vi "KeepWarm.vi"() -> ()   [LabVIEW 2010]
panel:
  in  "Current (mA)":dbl
  out "Dummy":string
  in  "Laser GPIB":u8=10 max=100
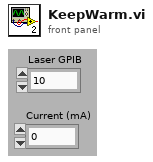
[diagram p1: front panel]
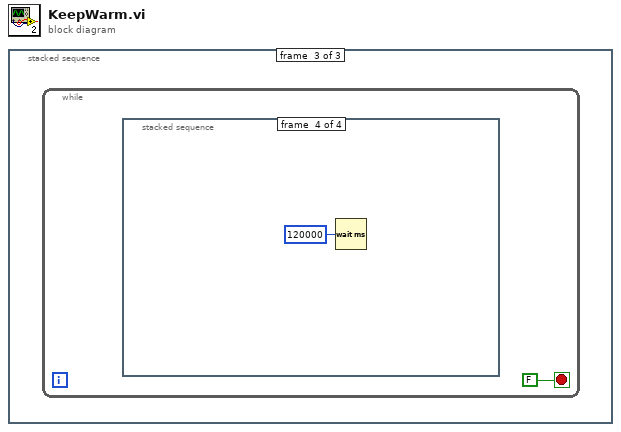
[diagram p0: block diagram]
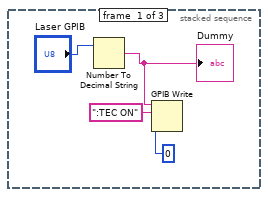
[diagram p2: hidden frame]
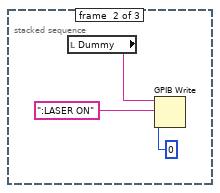
[diagram p3: hidden frame]
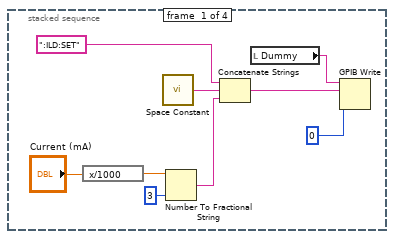
[diagram p4: hidden frame]
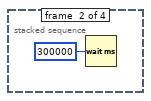
[diagram p5: hidden frame]
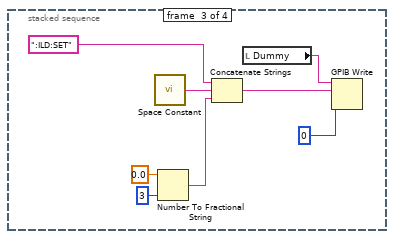
[diagram p6: hidden frame]
diagram:
  n1 = stacked-sequence {
    frame #0 {
      n2 = Number To Decimal String(number="Laser GPIB") -> (decimal integer string=w2:string)  [unwired: 1 in]
      "Dummy" <- w2
      n3 = GPIB Write(0:w2, 1:":TEC ON" ("data"), 2:i16 0 ("mode (0)")) -> ()  [unwired: 2 in, 2 out]
    }
    frame #1 {
      n4 = local read "Dummy"() -> (w6:string)
      n5 = GPIB Write(0:w6, 1:":LASER ON" ("data"), 2:i16 0 ("mode (0)")) -> ()  [unwired: 2 in, 2 out]
    }
    frame #2 {
      n6 = while {
        stop <- FALSE stop-if-true
        n7 = stacked-sequence {
          frame #0 {
            n8 = expression code="x/1000"("Current (mA)") -> (w9:dbl)
            n9 = call <vilib>:"Space Constant.vi"() -> ("String"=w14:string)
            n10 = Number To Fractional String(number=w9, precision (6)=i16 3) -> (F-format string=w12:string)  [unwired: 2 in]
            n11 = Concatenate Strings(":ILD:SET", w14, w12) -> (w15:string)
            n12 = local read "Dummy"() -> (w16:string)
            n13 = GPIB Write(0:w16, 1:w15, 2:i16 0 ("mode (0)")) -> ()  [unwired: 2 in, 2 out]
          }
          frame #1 {
            n14 = Wait (ms)(milliseconds to wait=u32 300000) -> ()  [unwired: 1 out]
          }
          frame #2 {
            n15 = call <vilib>:"Space Constant.vi"() -> ("String"=w22:string)
            n16 = Number To Fractional String(number=0.0, precision (6)=i16 3) -> (F-format string=w20:string)  [unwired: 2 in]
            n17 = Concatenate Strings(":ILD:SET", w22, w20) -> (w23:string)
            n18 = local read "Dummy"() -> (w24:string)
            n19 = GPIB Write(0:w24, 1:w23, 2:i16 0 ("mode (0)")) -> ()  [unwired: 2 in, 2 out]
          }
          frame #3 {
            n20 = Wait (ms)(milliseconds to wait=u32 120000) -> ()  [unwired: 1 out]
          }
        }
      }
    }
  }
